vi "GetFrontPanel.vi"(8 "Error In":errorcluster, 11 "object in":refnum<class "FlexPanelDefault.lvclass">) -> (0 "Error Out":errorcluster, 2 "FrontPanel":refnum<class "FrontPanelControl.lvclass">, 3 "object out":refnum<class "FlexPanelDefault.lvclass">)   [LabVIEW 2021, in "FlexPanelDefault.lvclass"]
uses:
  FlexPanelDefault.lvclass
  .Externals/Library_UserInterface_FrontPanelControl/FrontPanelControl/FrontPanelControl.lvclass
panel:
  # "Startup Screen\nof the \nApplication"
  # "Nice spot for an image :)"
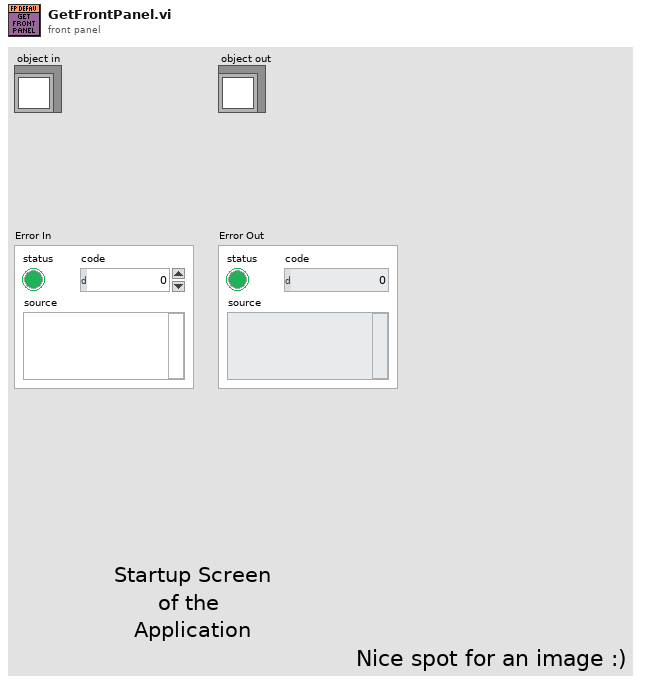
[diagram p1: front panel]
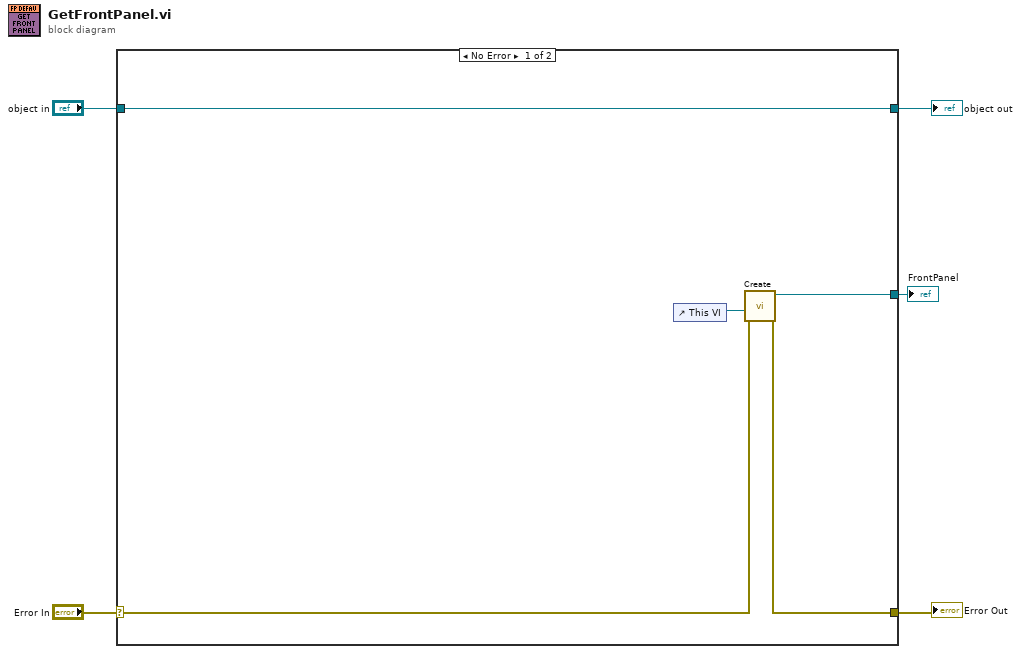
[diagram p0: block diagram]
diagram:
  n1 = case shown="No Error" "Error In" {
    selector: "Error In" -> [w7 w12]
    tunnel: [w6 w12] -> w4
    tunnel: [w10 w11] -> w2
    tunnel: "object in" -> [w10 w11]
    tunnel: [w8 _] -> w1
    frame No Error {
      n2 = control-ref of="This VI"() -> (w9:refnum<vi>)
      n3 = call "Create.vi"("ErrorIn"=w7, "VIRef"=w9) -> ("ErrorOut"=w6:errorcluster, "ObjectOut"=w8:refnum<class "FrontPanelControl.lvclass">)  [unwired: 8 in]
    }
    frame Error {
    }
  }
  "Error Out" <- w4
  "object out" <- w2
  "FrontPanel" <- w1
